vi "array dimension arry - scalar template.vi"() -> ()   [LabVIEW 2018]
panel:
  out "Array Size":i32[](array[numeric])
  in  "Numeric":dbl
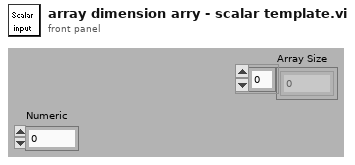
[diagram p1: front panel]
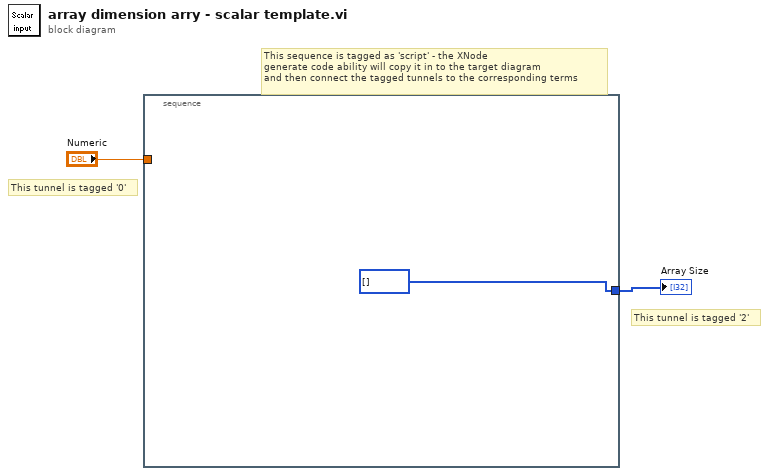
[diagram p0: block diagram]
diagram:
  # "This tunnel is tagged '2'"
  # "This tunnel is tagged '0'"
  # "This sequence is tagged as 'script' - the XNode \ngenerate code ability will copy it in to the target diagram\nand then connect the tagged tunnels to the corresponding terms"
  n1 = stacked-sequence {
    tunnel: "Numeric" -> [_]
    tunnel: [i32[] []] -> w1
    frame #0 {
    }
  }
  "Array Size" <- w1
